vi "Get NHMFL Synth Object.vi"() -> (3 "Module":refnum<class "Template Module.lvclass">)   [LabVIEW 2016]
uses:
  Template Module/Template Module.lvclass
  NHMFL Synthesizer.lvclass
  C:/github/LabActor/Template Module/Template Module.lvclass
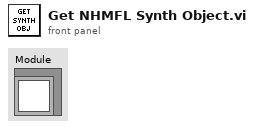
[diagram p1: front panel]
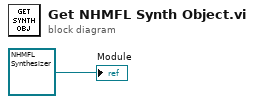
[diagram p0: block diagram]
diagram:
  "Module" <- refnum<class "NHMFL Synthesizer.lvclass"> refnum ("NHMFL Synthesizer.lvclass")
